vi "Script.vi"() -> ()   [LabVIEW 2020]
panel:
  in  "Data Source List":string(tree)
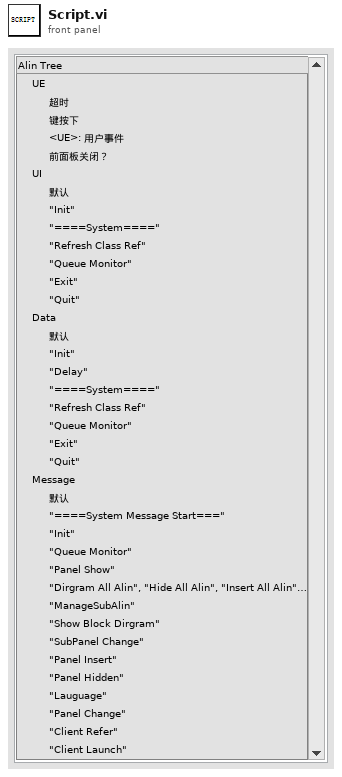
[diagram p1: front panel]
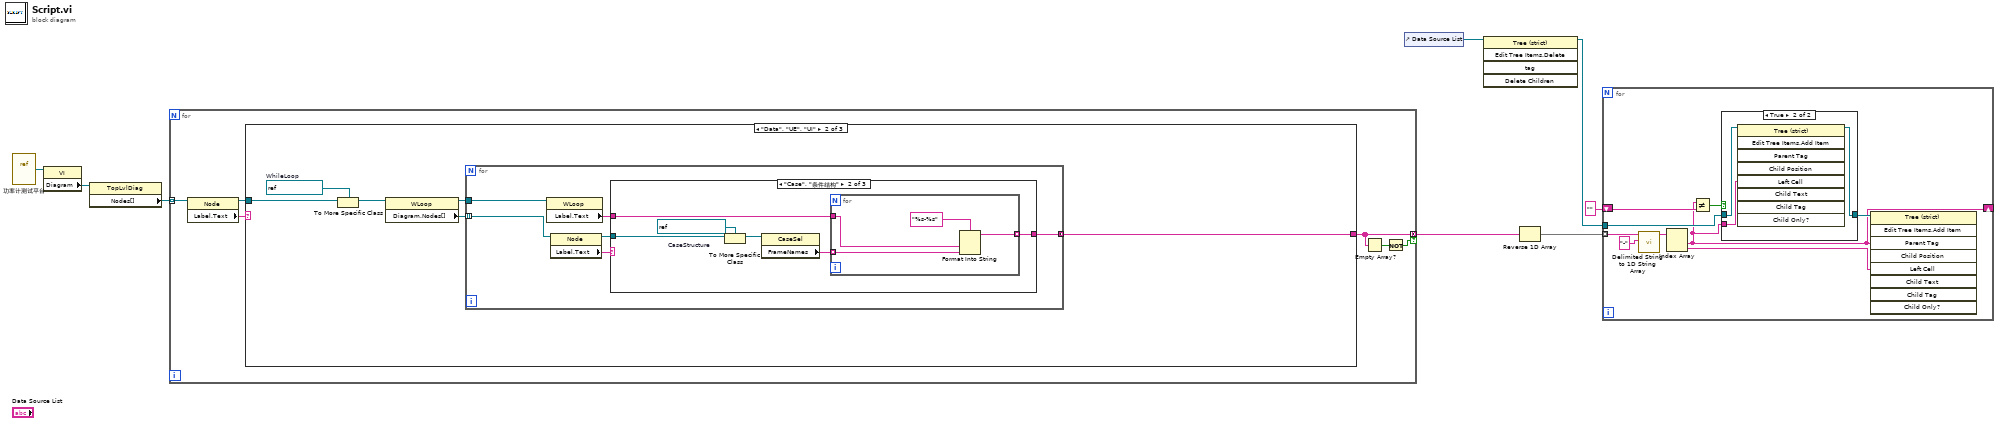
[diagram p0: block diagram]
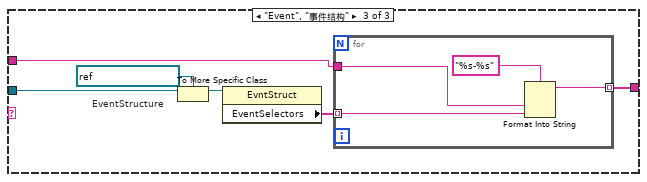
[diagram p5: hidden frame]
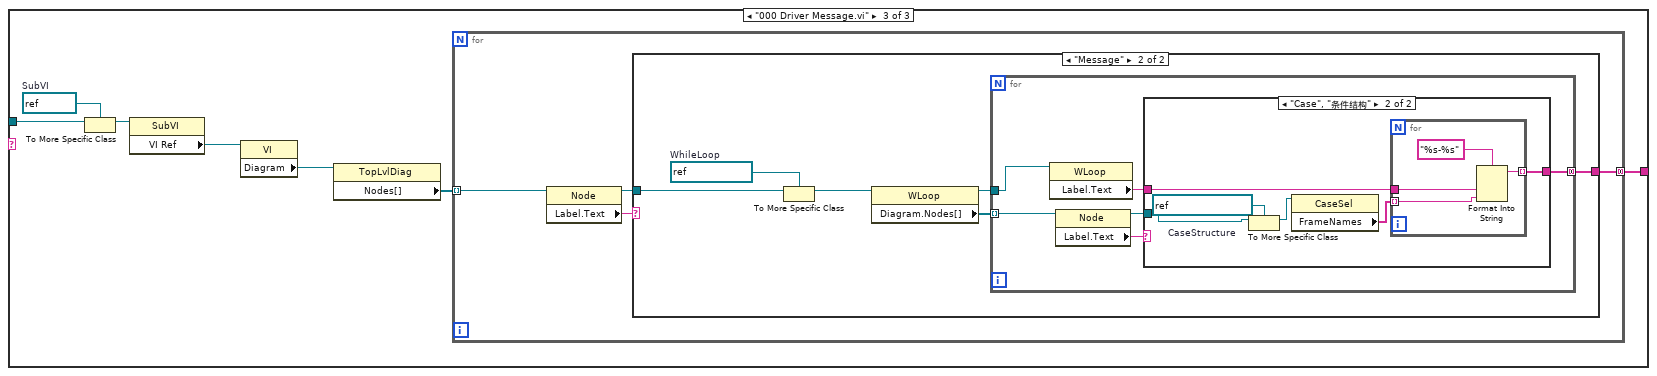
[diagram p6: hidden frame]
diagram:
  n1 = vi-ref "功率计测试平台.vi"() -> (w8:refnum<vi>)
  n2 = property class="VI"(reference=w8) -> ("Diagram"=w7:refnum<vi>)  [unwired: 1 in, 2 out]
  n3 = property class="TopLvlDiag"(reference=w7) -> ("Nodes[]"=w6:refnum<vi>[])  [unwired: 1 in, 2 out]
  n4 = for {
    tunnel: w6 -> [w14] mode=indexing
    tunnel: [w10] -> w5 mode=concatenating if=w9
    n5 = property class="Node"(reference=w14) -> (reference out=w12:refnum<vi>, "Label.Text"=w13:string)  [unwired: 1 in, 1 out]
    n6 = case shown="\"Data\", \"UE\", \"UI\"" w13 {
      tunnel: w12 -> [_ w20 w53]
      tunnel: [_ w15 w47] -> w10
      frame Default {
      }
      frame "Data", "UE", "UI" {
        w18 = refnum<vi> refnum  # WhileLoop
        n7 = To More Specific Class(target class=w18, reference=w20) -> (specific class reference=w19:refnum<vi>)  [unwired: 1 in, 1 out]
        n8 = property class="WLoop"(reference=w19) -> (reference out=w16:refnum<vi>, "Diagram.Nodes[]"=w17:refnum<vi>[])  [unwired: 1 in, 1 out]
        n9 = for {
          tunnel: w17 -> [w26] mode=indexing
          tunnel: w16 -> [w22]
          tunnel: [w23] -> w15 mode=concatenating
          n10 = property class="WLoop"(reference=w22) -> ("Label.Text"=w21:string)  [unwired: 1 in, 2 out]
          n11 = property class="Node"(reference=w26) -> (reference out=w24:refnum<vi>, "Label.Text"=w25:string)  [unwired: 1 in, 1 out]
          n12 = case shown="\"Case\", \"条件结构\"" w25 {
            tunnel: w24 -> [_ w31 w42]
            tunnel: [_ w28 w37] -> w23
            tunnel: w21 -> [_ w27 w38]
            frame Default {
            }
            frame "Case", "条件结构" {
              w32 = refnum<vi> refnum  # CaseStructure
              n13 = To More Specific Class(target class=w32, reference=w31) -> (specific class reference=w30:refnum<vi>)  [unwired: 1 in, 1 out]
              n14 = property class="CaseSel"(reference=w30) -> ("FrameNames"=w29:string[])  [unwired: 1 in, 2 out]
              n15 = for {
                tunnel: w29 -> [w35] mode=indexing
                tunnel: [w34] -> w28 mode=indexing
                tunnel: w27 -> [w33]
                n16 = Format Into String(format string="%s-%s" ("格式字符串"), w33, w35) -> (resulting string=w34:string)  [unwired: 2 in, 1 out]
              }
            }
            frame "Event", "事件结构" {
              w41 = refnum<vi> refnum  # EventStructure
              n17 = To More Specific Class(target class=w41, reference=w42) -> (specific class reference=w40:refnum<vi>)  [unwired: 1 in, 1 out]
              n18 = property class="EvntStruct"(reference=w40) -> ("EventSelectors"=w39:string[])  [unwired: 1 in, 2 out]
              n19 = for {
                tunnel: w39 -> [w45] mode=indexing
                tunnel: w38 -> [w44]
                tunnel: [w43] -> w37 mode=indexing
                n20 = Format Into String(format string="%s-%s" ("格式字符串"), w44, w45) -> (resulting string=w43:string)  [unwired: 2 in, 1 out]
              }
            }
          }
        }
      }
      frame "000 Driver Message.vi" {
        w52 = refnum<vi> refnum  # SubVI
        n21 = To More Specific Class(target class=w52, reference=w53) -> (specific class reference=w51:refnum<vi>)  [unwired: 1 in, 1 out]
        n22 = property class="SubVI"(reference=w51) -> ("VI Ref"=w49:refnum<vi>)  [unwired: 1 in, 2 out]
        n23 = property class="VI"(reference=w49) -> ("Diagram"=w50:refnum<vi>)  [unwired: 1 in, 2 out]
        n24 = property class="TopLvlDiag"(reference=w50) -> ("Nodes[]"=w48:refnum<vi>[])  [unwired: 1 in, 2 out]
        n25 = for {
          tunnel: w48 -> [w57] mode=indexing
          tunnel: [w54] -> w47 mode=concatenating
          n26 = property class="Node"(reference=w57) -> (reference out=w55:refnum<vi>, "Label.Text"=w56:string)  [unwired: 1 in, 1 out]
          n27 = case shown="\"Message\"" w56 {
            tunnel: w55 -> [_ w61]
            tunnel: [_ w58] -> w54
            frame Default {
            }
            frame "Message" {
              w62 = refnum<vi> refnum  # WhileLoop
              n28 = To More Specific Class(target class=w62, reference=w61) -> (specific class reference=w63:refnum<vi>)  [unwired: 1 in, 1 out]
              n29 = property class="WLoop"(reference=w63) -> (reference out=w59:refnum<vi>, "Diagram.Nodes[]"=w60:refnum<vi>[])  [unwired: 1 in, 1 out]
              n30 = for {
                tunnel: w60 -> [w69] mode=indexing
                tunnel: w59 -> [w65]
                tunnel: [w66] -> w58 mode=concatenating
                n31 = property class="WLoop"(reference=w65) -> ("Label.Text"=w64:string)  [unwired: 1 in, 2 out]
                n32 = property class="Node"(reference=w69) -> (reference out=w67:refnum<vi>, "Label.Text"=w68:string)  [unwired: 1 in, 1 out]
                n33 = case shown="\"Case\", \"条件结构\"" w68 {
                  tunnel: w67 -> [_ w74]
                  tunnel: [_ w71] -> w66
                  tunnel: w64 -> [_ w70]
                  frame Default {
                  }
                  frame "Case", "条件结构" {
                    w75 = refnum<vi> refnum  # CaseStructure
                    n34 = To More Specific Class(target class=w75, reference=w74) -> (specific class reference=w73:refnum<vi>)  [unwired: 1 in, 1 out]
                    n35 = property class="CaseSel"(reference=w73) -> ("FrameNames"=w72:string[])  [unwired: 1 in, 2 out]
                    n36 = for {
                      tunnel: w72 -> [w78] mode=indexing
                      tunnel: [w77] -> w71 mode=indexing
                      tunnel: w70 -> [w76]
                      n37 = Format Into String(format string="%s-%s" ("格式字符串"), w76, w78) -> (resulting string=w77:string)  [unwired: 2 in, 1 out]
                    }
                  }
                }
              }
            }
          }
        }
      }
    }
    n38 = Empty Array?(array=w10) -> (empty?=w11:bool)
    n39 = Not(x=w11) -> (.not. x?=w9:bool)
  }
  n40 = control-ref of="Data Source List"() -> (w4:refnum<vi>)
  n41 = invoke class="Tree (strict)" method="Edit Tree Items.Delete"(reference=w4) -> (reference out=w3:refnum<vi>)  [unwired: 4 in, 4 out]
  n42 = Reverse 1D Array(array=w5) -> (reversed array=w2:string[])
  n43 = for {
    tunnel: w2 -> [w88] mode=indexing
    tunnel: w3 -> [w84]
    shift-right: [w80] -> _
    shift-left: "" ("元素") -> [w85]
    n44 = call <vilib>:"Delimited String to 1D String Array.vi"("delimiter"="-", "delimited string"=w88) -> ("string array"=w86:string[])  [unwired: 9 in]
    n45 = Index Array(array=w86) -> (element #1=w80:string, element #2=w81:string)  [unwired: 2 in]
    n46 = Not Equal?(x=w80, y=w85) -> (x != y?=w82:bool)
    n47 = case shown="True" w82 {
      tunnel: w84 -> [w89 w92]
      tunnel: [w89 w91] -> w83
      tunnel: w80 -> [_ w90]
      frame False {
      }
      frame True {
        n48 = invoke class="Tree (strict)" method="Edit Tree Items.Add Item"(reference=w92, "Left Cell"=w90) -> (reference out=w91:refnum<vi>)  [unwired: 7 in, 8 out]
      }
    }
    n49 = invoke class="Tree (strict)" method="Edit Tree Items.Add Item"(reference=w83, "Parent Tag"=w80, "Left Cell"=w81) -> ()  [unwired: 6 in, 9 out]
  }
